vi "Copy of IMAQ HL-Snap.vi"(7 "ImgName":string="untitled", 8 "ErrIn":errorcluster, 11 "IF Name":string="img0") -> (0 "ErrOut":errorcluster, 3 "ImgOut":T1)   [LabVIEW 2016]
doc: "Use this template to build a VI to use as a subVI."
uses:
  <vilib>/vision/Image Controls.llb/IMAQ Image.ctl
panel:
  out "SubValue":dbl
  out "Value":string
  # "Input Parameters"
  # "Output Parameters"
  # "VI Description:\nThis VI is created to snap a image from imaging device."
  # ":: MVI Framework V1.0 ::\nAuthor:Gaoke Yang\nEmail: gaoke.yang@yahoo.com\nWeb: www.mvicontrol.com\nCopyright (C) , MVI Technologies All Rights Reserved"
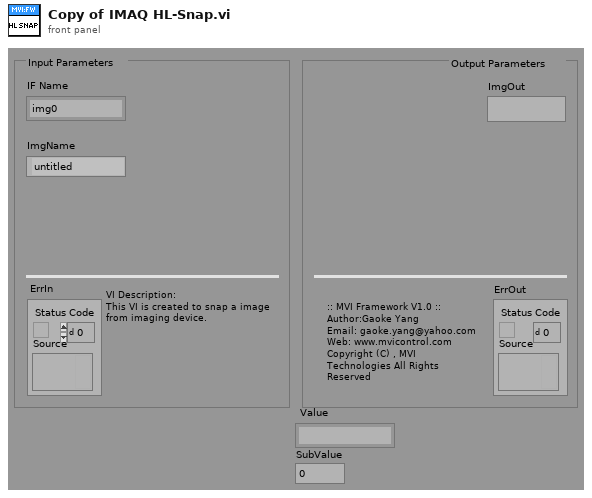
[diagram p1: front panel]
types:
  T1 = typedef "IMAQ Image.ctl" = refnum<image>
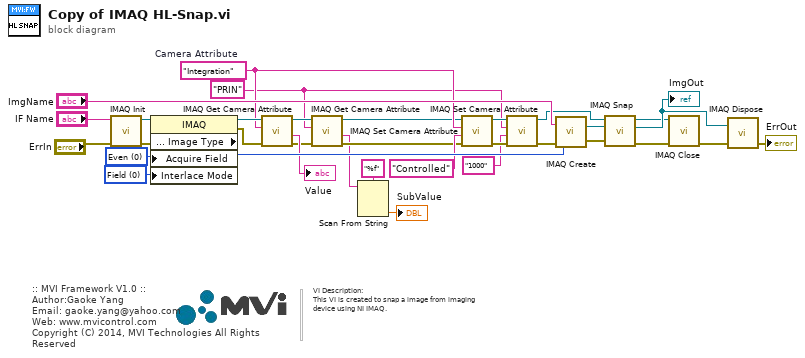
[diagram p0: block diagram]
diagram:
  w4 = "PRIN" ("Camera Attribute")
  w11 = "Integration"  # Camera Attribute
  w19 = 0 items=["Field", "Frame"] ("Image Parameters : Interlacing : Mode")
  w20 = 0 items=["Even", "Odd", "All"] ("Image Parameters : Interlacing : Acquire Field")
  # "VI Description:\nThis VI is created to snap a image from imaging\ndevice using NI IMAQ."
  # ":: MVI Framework V1.0 ::\nAuthor:Gaoke Yang\nEmail: gaoke.yang@yahoo.com\nWeb: www.mvicontrol.com\nCopyright (C) 2014, MVI Technologies All Rights Reserved"
  n1 = call <vilib>:"IMAQ Init.vi"("error in (no error)"="ErrIn", "Interface Name"="IF Name") -> ("error out"=w26:errorcluster, "IMAQ Session Out"=w27:refnum<k11>)  [unwired: 8 out]
  n2 = property class="IMAQ"(reference=w27, error in=w26, "Acquire Field"=w20, "Interlace Mode"=w19) -> (reference out=w18:refnum<k11>, error out=w17:errorcluster, "Image Parameters : Image Type"=w25:u32)
  n3 = call <vilib>:"IMAQ Get Camera Attribute.vi"("error in (no error)"=w17, "Camera Attribute"=w11, "IMAQ Session In"=w18) -> ("error out"=w7:errorcluster, "Attribute Value"=→"Value":string, "IMAQ Session Out"=w8:refnum<k11>)  [unwired: 4 in]
  n4 = call <vilib>:"IMAQ Get Camera Attribute.vi"("error in (no error)"=w7, "Camera Attribute"=w4, "IMAQ Session In"=w8) -> ("error out"=w5:errorcluster, "Attribute Value"=w2:string, "IMAQ Session Out"=w6:refnum<k11>)  [unwired: 4 in]
  n5 = Scan From String(format string="%f", input string=w2) -> (output 1=→"SubValue":dbl)  [unwired: 3 in, 3 out]
  n6 = call <vilib>:"IMAQ Set Camera Attribute.vi"("error in (no error)"=w5, "Attribute Value"="Controlled", "Camera Attribute"=w11, "IMAQ Session In"=w6) -> ("error out"=w16:errorcluster, "IMAQ Session Out"=w15:refnum<k11>)  [unwired: 4 in]
  n7 = call <vilib>:"IMAQ Set Camera Attribute.vi"("error in (no error)"=w16, "Attribute Value"="1000", "Camera Attribute"=w4, "IMAQ Session In"=w15) -> ("error out"=w13:errorcluster, "IMAQ Session Out"=w14:refnum<k11>)  [unwired: 4 in]
  n8 = call "IMAQ Create"("Image Name"="ImgName", "Image Type"=w25, "error in (no error)"=w13) -> ("New Image"=w28:T1, "error out"=w24:errorcluster)  [unwired: 1 in, 1 out]
  n9 = call <vilib>:"IMAQ Snap.vi"("error in (no error)"=w24, "Image In"=w28, "IMAQ Session In"=w14) -> ("error out"=w21:errorcluster, "Image Out"=w29:T1, "IMAQ Session Out"=w22:refnum<k11>)  [unwired: 6 out]
  "ImgOut" <- w29
  n10 = call <vilib>:"IMAQ Close.vi"("error in (no error)"=w21, "IMAQ Session In"=w22) -> ("error out"=w23:errorcluster)  [unwired: 9 out]
  n11 = call "IMAQ Dispose"("Image"=w29, "error in (no error)"=w23) -> ("error out"=→"ErrOut":errorcluster)  [unwired: 1 in, 3 out]
